vi "Streaming - Write.vi"() -> ()   [LabVIEW 2020]
uses:
  Nominal Client/Nominal Client.lvclass/Nominal Client.ctl
  68912467-c1c9-4a94-a3ad-dccbebf4617c.vi
  6412a388-4fe4-4984-8121-4c3d8e6ce4ff.vi
  8bc873d6-11f2-47b8-afa9-2ee06eb45ce7.vi
  6412a388-4fe4-4984-8121-4c3d8e6ce4ff.vi/028fdd67-09da-40c6-8995-0c4bd62a0b31.vi
  <vilib>/JDP Science/JSONtext/Make JSON Object.vi
  6412a388-4fe4-4984-8121-4c3d8e6ce4ff.vi/c2a1aca9-ea5a-4b2a-8072-18de54756c53.vi
  <vilib>/JDP Science/JSONtext/Make JSON Array.vi
  6412a388-4fe4-4984-8121-4c3d8e6ce4ff.vi/2c8a2fb0-06af-4bda-9dcc-d72a85547e70.vi
  Nominal Client/private_data.set.vi
  <vilib>/LabVIEW Open Source Project/Epoch Date & Time/epoch.UNIX/Epoch.UNIX.lvclass
  C:/Program Files/National Instruments/LabVIEW 2020/vi.lib/LabVIEW Open Source Project/Epoch Date & Time/epoch/Epoch.lvclass
  <vilib>/Utility/file.llb/Application Directory.vi
  <vilib>/Utility/error.llb/Error Cluster From Error Code.vi
  submodules/reqwest-labview/lv-src/reqwest/create.vi
  <vilib>/LabVIEW Open Source Project/Epoch Date & Time/Get Epoch Time.vi
  nominal types/properties/create.from_map.vi
  Nominal Client/nominal_channel_writer.write_batches.path.vi
  <vilib>/JDP Science/JSONtext/Variant to JSON Text.vi
  <vilib>/JDP Science/JSONtext/support/Format JSON Object.vi
  <vilib>/JDP Science/JSONtext/support/Format JSON Array Text.vi
  Nominal Client/http.post.vi
  Nominal Client/Nominal Client.lvclass
  nominal types/workspace/workspace.lvclass
  submodules/reqwest-labview/lv-src/reqwest/reqwest.lvclass
  <vilib>/JDP Science/JSONtext/LVClass Serializer/JSONtext LVClass Serializer.lvclass
  nominal types/properties/properties.lvclass
panel:
  in  "API Token":string
  in  "Data Source RID":string
  in  "Stop":bool
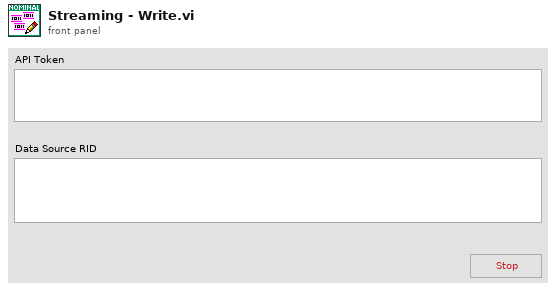
[diagram p1: front panel]
types:
  T1 = cluster{"channel":string, "current time":timestamp, "data":dbl}
  T2 = cluster{"[0]":refnum<queue>, "[1]":refnum<queue>, "[2]":refnum<queue>}
  T3 = cluster{"channel":string, "current time":timestamp, "data":dbl}[]
  T4 = cluster{"UNIX Timestamp":cluster{"Seconds":i64, "Nanoseconds":i64}, "data":dbl}
  T5 = cluster{"channel":string, cluster{"UNIX Timestamp":cluster{"Seconds":i64, "Nanoseconds":i64}, "data":dbl}[]}
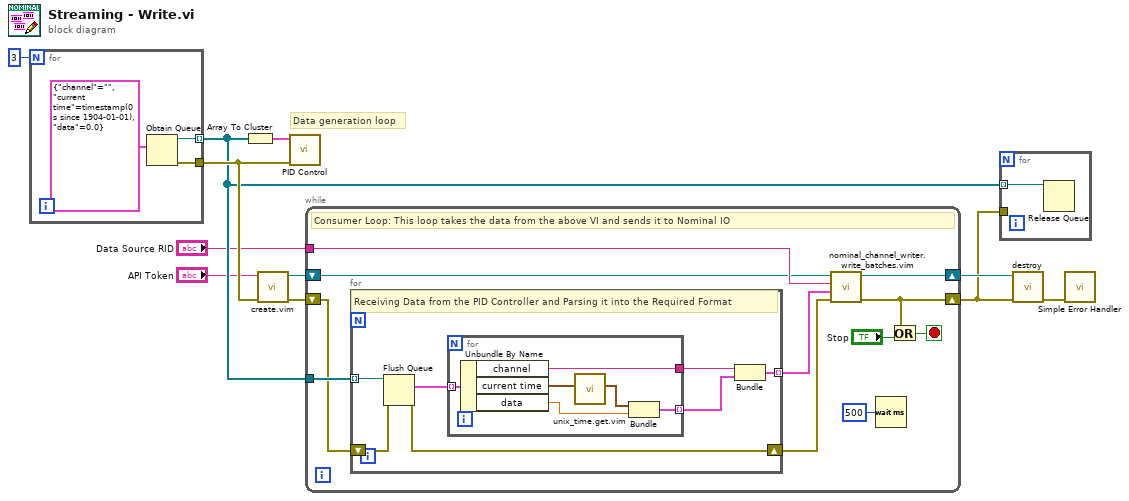
[diagram p0: block diagram]
diagram:
  # "Data generation loop"
  n1 = for {
    N: 3 -> [_]
    tunnel: [w13] -> w4 mode=indexing
    tunnel: [w12] -> w8
    n2 = Obtain Queue(element data type=T1 {"channel"="", "current time"=timestamp(0 s since 1904-01-01), "data"=0.0}) -> (queue out=w13:refnum<queue>, error out=w12:errorcluster)  [unwired: 4 in, 1 out]
  }
  n3 = Array To Cluster(array=w4) -> (cluster=w5:T2)
  n4 = call "create.vim"("error in"=w8, "API Token (string or path)"="API Token") -> ("error out"=w9:errorcluster, "Nominal Client"=w10:refnum<class "Nominal Client.lvclass">)  [unwired: 8 in]
  n5 = call "PID Control.vi"("error in (no error)"=w8, "Data"=w5) -> ()  [unwired: 10 in]
  n6 = while {
    tunnel: w4 -> [w22]
    shift-right: [w19] -> w3
    shift-left: w9 -> [w21]
    shift-right: [w20] -> w11
    shift-left: w10 -> [w17]
    tunnel: "Data Source RID" -> [w18]
    stop <- w24 stop-if-true
    # "Consumer Loop: This loop takes the data from the above VI and sends it to Nominal IO"
    n7 = for {
      tunnel: w22 -> [w32] mode=indexing
      tunnel: [w28] -> w15 mode=indexing
      shift-right: [w26] -> w16
      shift-left: w21 -> [w27]
      # "Receiving Data from the PID Controller and Parsing it into the Required Format"
      n8 = Flush Queue(queue=w32, error in (no error)=w27) -> (remaining elements=w31:T3, error out=w26:errorcluster)  [unwired: 1 out]
      n9 = for {
        tunnel: w31 -> [w38] mode=indexing
        tunnel: [w34] -> w29 mode=indexing
        tunnel: [w33] -> w30
        n10 = Unbundle By Name(w38) -> ("channel"=w33:string, "current time"=w37:timestamp, "data"=w35:dbl)
        n11 = call "unix_time.get.vim"("Time Stamp (empty: now) [single or array]"=w37) -> ("UNIX Timestamp"=w36:cluster{"Seconds":i64, "Nanoseconds":i64})  [unwired: 10 in]
        n12 = Bundle("UNIX Timestamp"=w36, "data"=w35) -> (w34:T4)  [unwired: 1 in]
      }
      n13 = Bundle("channel"=w30, w29) -> (w28:T5)  [unwired: 1 in]
    }
    n14 = call "nominal_channel_writer.write_batches.vim"("error in"=w16, "batches"=w15, "Data Source RID"=w18, "Nominal Client in"=w17) -> ("error out"=w19:errorcluster, "Nominal Client out"=w20:refnum<class "Nominal Client.lvclass">)  [unwired: 5 in, 1 out]
    n15 = Wait (ms)(milliseconds to wait=u32 500) -> ()  [unwired: 1 out]
    n16 = Or(x=w19, y="Stop") -> (x .or. y?=w24:bool)
  }
  n17 = for {
    tunnel: w4 -> [w39] mode=indexing
    tunnel: w3 -> [_]
    n18 = Release Queue(queue=w39) -> ()  [unwired: 2 in, 3 out]
  }
  n19 = call "destroy.vi"("error in"=w3, "Nominal Client"=w11) -> ("error out"=w7:errorcluster)  [unwired: 9 in]
  n20 = call <vilib>:"Simple Error Handler.vi"("error in (no error)"=w7) -> ()  [unwired: 4 in, 5 out]
